vi "Query Setpoint Limits.vi"(7 "Channel (0: Channel A)":u16(ring) items=["Channel A", "Channel B"], 8 "error in (no error)":errorcluster, 11 "BH Druck PACE Series in":refnum<class "BH Druck PACE Series.lvclass">) -> (0 "error out":errorcluster, 1 "Lower Setpoint Limit":dbl, 2 "Upper Setpoint Limit":dbl, 3 "BH Druck PACE Series out":refnum<class "BH Druck PACE Series.lvclass">)   [LabVIEW 2022 SP3, in "BH Druck PACE Series.lvclass"]
uses:
  BH Druck PACE Series.lvclass
  BH Druck PACE Series.lvclass/BH Druck PACE Series.ctl
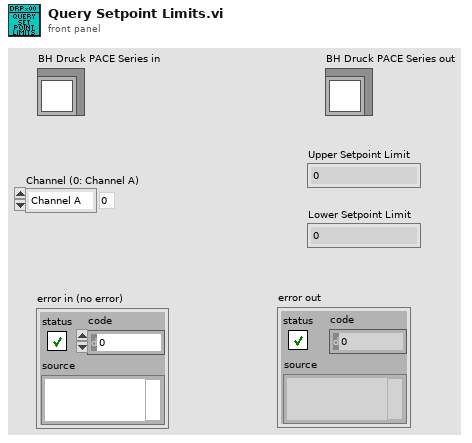
[diagram p1: front panel]
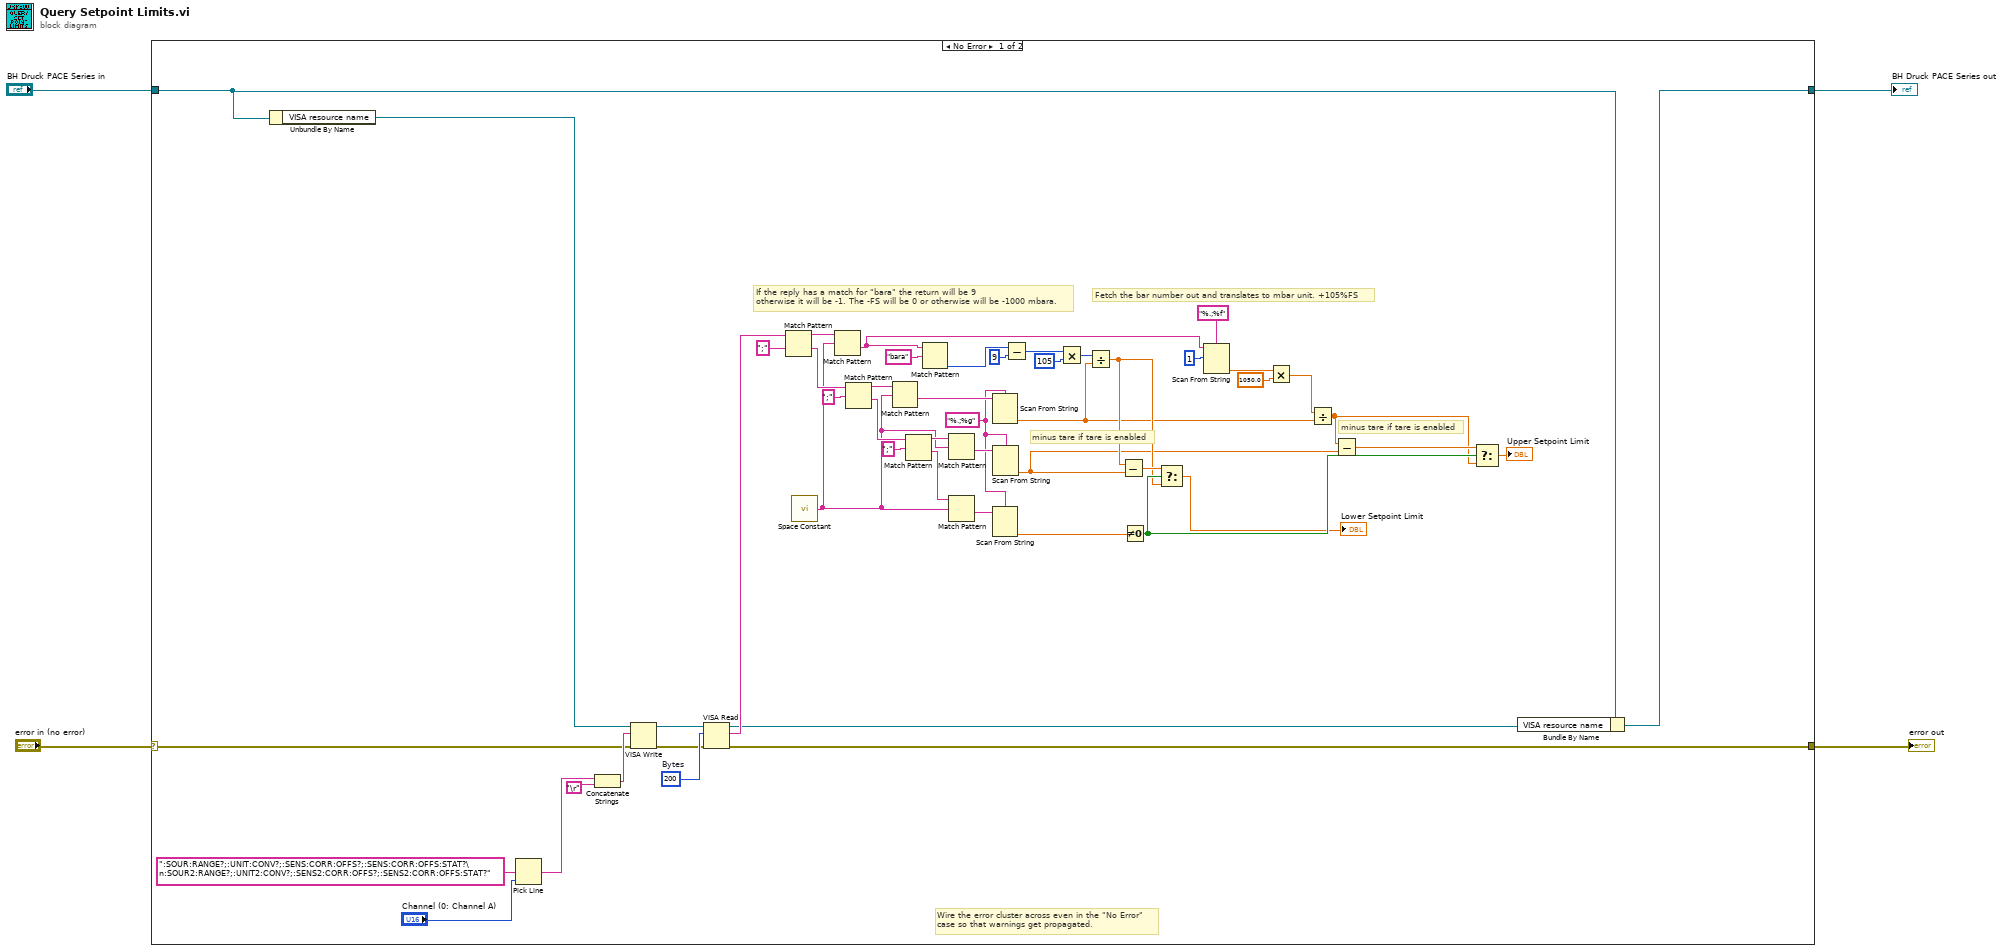
[diagram p0: block diagram]
diagram:
  n1 = case shown="No Error" "error in (no error)" {
    selector: "error in (no error)" -> [w10 w57]
    tunnel: [w8 w57] -> w3
    tunnel: [w5 w56] -> w1
    tunnel: "BH Druck PACE Series in" -> [w7 w56]
    frame No Error {
      w34 = "%.;%g" ("Format String")
      w52 = u32 200  # Bytes
      # "Wire the error cluster across even in the \"No Error\"\ncase so that warnings get propagated."
      # "minus tare if tare is enabled"
      # "minus tare if tare is enabled"
      # "Fetch the bar number out and translates to mbar unit. +105%FS"
      # "If the reply has a match for \"bara\" the return will be 9 \notherwise it will be -1. The -FS will be 0 or otherwise will be -1000 mbara."
      n2 = Unbundle By Name(w7) -> ("VISA resource name"=w9:refnum<visa-resource-name>)
      n3 = Pick Line(multi-line string=":SOUR:RANGE?;:UNIT:CONV?;:SENS:CORR:OFFS?;:SENS:CORR:OFFS:STAT?\n:SOUR2:RANGE?;:UNIT2:CONV?;:SENS2:CORR:OFFS?;:SENS2:CORR:OFFS:STAT?", line index="Channel (0: Channel A)") -> (output string=w48:string)  [unwired: 1 in]
      n4 = Concatenate Strings(w48, "\r" ("Carriage Return Constant")) -> (w46:string)
      n5 = VISA Write(VISA resource name=w9, write buffer=w46, error in (no error)=w10) -> (VISA resource name out=w50:refnum<visa-resource-name>, error out=w51:errorcluster)  [unwired: 1 out]
      n6 = VISA Read(VISA resource name=w50, byte count=w52, error in (no error)=w51) -> (VISA resource name out=w6:refnum<visa-resource-name>, read buffer=w47:string, error out=w8:errorcluster)  [unwired: 1 out]
      n7 = Match Pattern(string=w47, regular expression=";") -> (before substring=w45:string, after substring=w42:string)  [unwired: 1 in, 2 out]
      n8 = call <vilib>:"Space Constant.vi"() -> ("String"=w33:string)
      n9 = Match Pattern(string=w45, regular expression=w33) -> (after substring=w12:string)  [unwired: 1 in, 3 out]
      n10 = Match Pattern(string=w42, regular expression=";") -> (before substring=w39:string, after substring=w40:string)  [unwired: 1 in, 2 out]
      n11 = Match Pattern(string=w39, regular expression=w33) -> (after substring=w44:string)  [unwired: 1 in, 3 out]
      n12 = Match Pattern(string=w40, regular expression=";") -> (before substring=w37:string, after substring=w35:string)  [unwired: 1 in, 2 out]
      n13 = Match Pattern(string=w12, regular expression="bara") -> (offset past match=w27:i32)  [unwired: 1 in, 3 out]
      n14 = Match Pattern(string=w37, regular expression=w33) -> (after substring=w38:string)  [unwired: 1 in, 3 out]
      n15 = Match Pattern(string=w35, regular expression=w33) -> (after substring=w36:string)  [unwired: 1 in, 3 out]
      n16 = Scan From String(format string=w34, input string=w44) -> (output 1=w11:dbl)  [unwired: 3 in, 3 out]
      n17 = Scan From String(format string=w34, input string=w36) -> (output 1=w14:dbl)  [unwired: 3 in, 3 out]
      n18 = Scan From String(format string=w34, input string=w38) -> (output 1=w13:dbl)  [unwired: 3 in, 3 out]
      n19 = Subtract(x=w27, y=9) -> (x-y=w25:i32)
      n20 = Multiply(x=w25, y=105) -> (x*y=w22:i32)
      n21 = Divide(x=w22, y=w11) -> (x/y=w17:dbl)
      n22 = Subtract(x=w17, y=w13) -> (x-y=w20:dbl)
      n23 = Not Equal To 0?(x=w14) -> (x != 0?=w19:bool)
      n24 = Select(t=w20, s=w19, f=w17) -> (s? t:f=→"Lower Setpoint Limit":dbl)
      n25 = Scan From String(format string="%.;%f", input string=w12, initial scan location=u32 1) -> (output 1=w30:dbl)  [unwired: 2 in, 3 out]
      n26 = Multiply(x=w30, y=1050.0) -> (x*y=w23:dbl)
      n27 = Divide(x=w23, y=w11) -> (x/y=w18:dbl)
      n28 = Subtract(x=w18, y=w13) -> (x-y=w21:dbl)
      n29 = Select(t=w21, s=w19, f=w18) -> (s? t:f=→"Upper Setpoint Limit":dbl)
      n30 = Bundle By Name(cluster=w7, "VISA resource name"=w6) -> (w5:refnum<class "BH Druck PACE Series.lvclass">)
    }
    frame Error {
    }
  }
  "error out" <- w3
  "BH Druck PACE Series out" <- w1
